vi "HTS_WELL_TO_#.vi"(1 "Well Array":T1[](array[typedef])) -> (0 "Position Array":i32[](array[numeric]))   [LabVIEW 2009]
uses:
  HTS_WELL.ctl
  HTS_COLUMN.ctl
  HTS_ROW.ctl
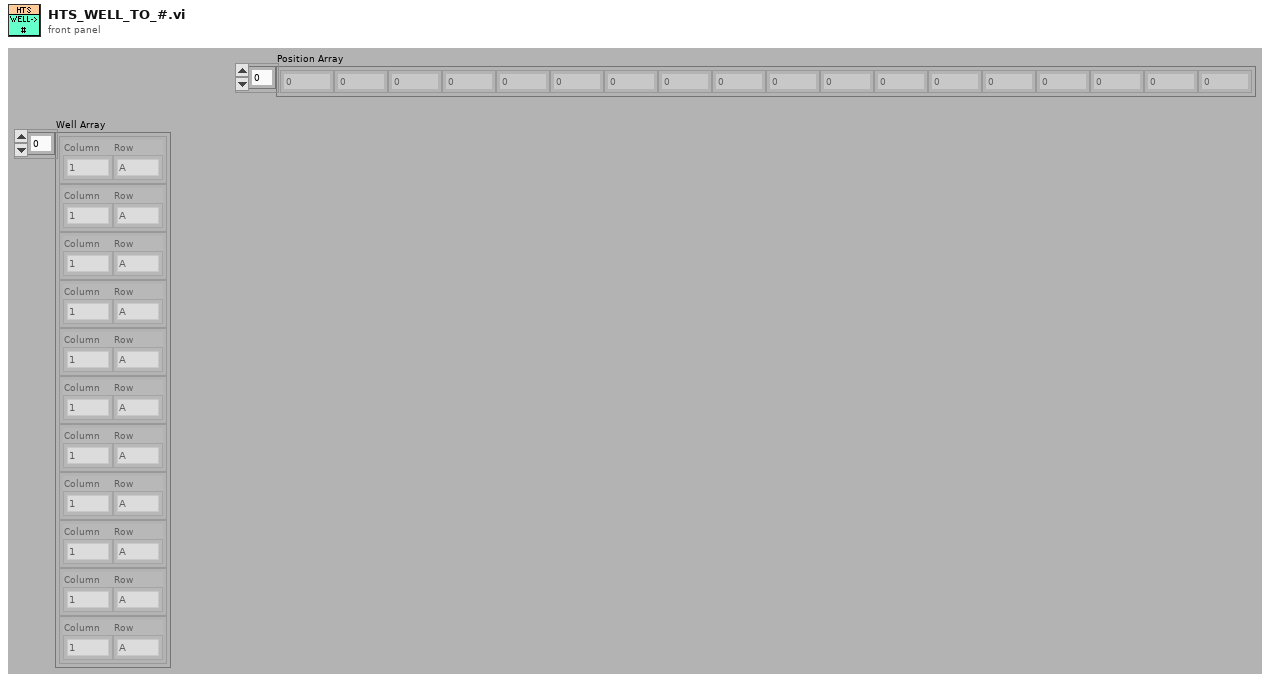
[diagram p1: front panel]
types:
  T1 = typedef "HTS_WELL.ctl" = cluster{"Column":T2, "Row":T3}
  T2 = typedef "HTS_COLUMN.ctl" = enum16{"1", "2", "3", "4", "5", "6", "7", "8", "9", "10", "11", "12"}
  T3 = typedef "HTS_ROW.ctl" = enum16{"A", "B", "C", "D", "E", "F", "G", "H"}
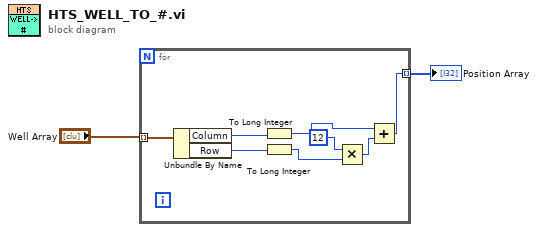
[diagram p0: block diagram]
diagram:
  n1 = for {
    tunnel: "Well Array" -> [w10] mode=indexing
    tunnel: [w3] -> w1 mode=indexing
    n2 = Unbundle By Name(w10) -> ("Column"=w8:T2, "Row"=w9:T3)
    n3 = To Long Integer(number=w8) -> (32bit integer=w5:i32)
    n4 = To Long Integer(number=w9) -> (32bit integer=w6:i32)
    n5 = Multiply(x=12 ("dimension size"), y=w6) -> (x*y=w4:i32)
    n6 = Add(x=w5, y=w4) -> (x+y=w3:i32)
  }
  "Position Array" <- w1
